vi "ui add or modify exif data.vi"() -> ()   [LabVIEW 2023]
panel:
  out "error":string
  out "Progress":string
  out "Error Array":string[](array[string])
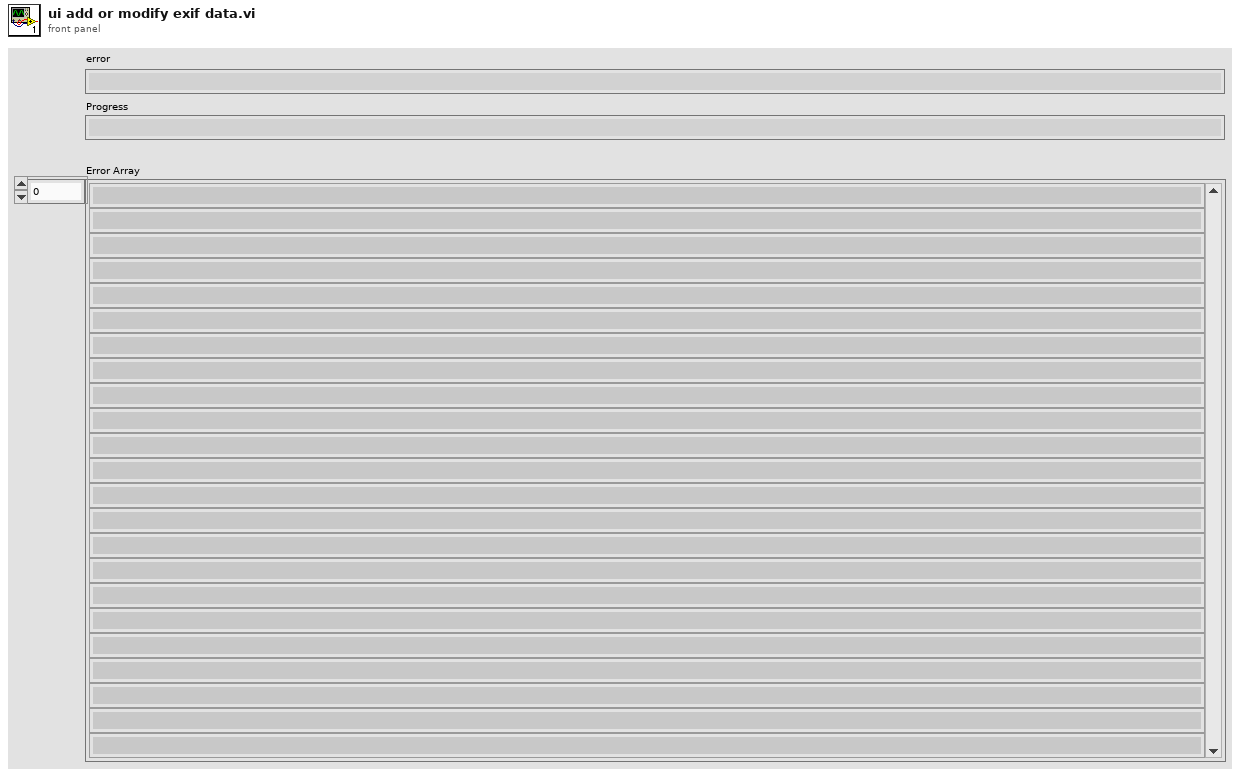
[diagram p1: front panel]
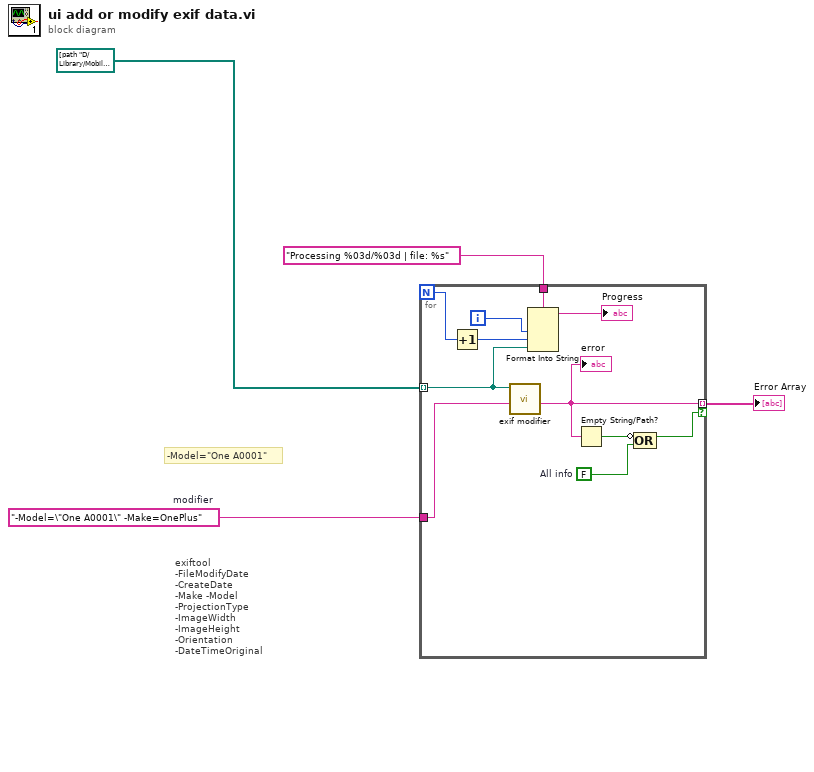
[diagram p0: block diagram]
diagram:
  w4 = "-Model=\"One A0001\" -Make=OnePlus"  # modifier
  # "-Model=\"One A0001\""
  # "exiftool \n-FileModifyDate \n-CreateDate \n-Make -Model \n-ProjectionType \n-ImageWidth \n-ImageHeight \n-Orientation \n-DateTimeOriginal"
  n1 = for {
    N -> [w10]
    tunnel: path[] [path "D:/Library/Mobile Repository/OnePlus1 Data/DNG Files/IMG_20160511_193852.dng", path "D:/Library/Mobile Repository/OnePlus1 Data/DNG Files/IMG_20160511_193916.dng", path "D:/Library/Mobile Repository/OnePlus1 Data/DNG Files/IMG_20160512_134053.dng", path "D:/Library/Mobile Repository/OnePlus1 Data/DNG Files/IMG_20160512_134058.dng", path "D:/Library/Mobile Repository/OnePlus1 Data/DNG Files/IMG_20160512_211940.dng", path "D:/Library/Mobile Repository/OnePlus1 Data/DNG Files/IMG_20160513_183751.dng", path "D:/Library/Mobile Repository/OnePlus1 Data/DNG Files/IMG_20160513_183754.dng", path "D:/Library/Mobile Repository/OnePlus1 Data/DNG Files/IMG_20160513_183809.dng", path "D:/Library/Mobile Repository/OnePlus1 Data/DNG Files/IMG_20160513_183823.dng", path "D:/Library/Mobile Repository/OnePlus1 Data/DNG Files/IMG_20160513_183826.dng", path "D:/Library/Mobile Repository/OnePlus1 Data/DNG Files/IMG_20160513_183840.dng", path "D:/Library/Mobile Repository/OnePlus1 Data/DNG Files/IMG_20160515_153030.dng", path "D:/Library/Mobile Repository/OnePlus1 Data/DNG Files/IMG_20160515_155700.dng", path "D:/Library/Mobile Repository/OnePlus1 Data/DNG Files/IMG_20160516_195620.dng", path "D:/Library/Mobile Repository/OnePlus1 Data/DNG Files/IMG_20160516_195635.dng", path "D:/Library/Mobile Repository/OnePlus1 Data/DNG Files/IMG_20160625_125528.dng", path "D:/Library/Mobile Repository/OnePlus1 Data/DNG Files/IMG_20160625_181705.dng", path "D:/Library/Mobile Repository/OnePlus1 Data/DNG Files/IMG_20160625_181731.dng", path "D:/Library/Mobile Repository/OnePlus1 Data/DNG Files/IMG_20160626_165512.dng", path "D:/Library/Mobile Repository/OnePlus1 Data/DNG Files/IMG_20160626_165517.dng", path "D:/Library/Mobile Repository/OnePlus1 Data/DNG Files/IMG_20160626_165523.dng", path "D:/Library/Mobile Repository/OnePlus1 Data/DNG Files/IMG_20160626_175208.dng", path "D:/Library/Mobile Repository/OnePlus1 Data/DNG Files/IMG_20160626_175216.dng", path "D:/Library/Mobile Repository/OnePlus1 Data/DNG Files/IMG_20160627_101057.dng", path "D:/Library/Mobile Repository/OnePlus1 Data/DNG Files/IMG_20160627_164656.dng", path "D:/Library/Mobile Repository/OnePlus1 Data/DNG Files/IMG_20160627_164716.dng", path "D:/Library/Mobile Repository/OnePlus1 Data/DNG Files/IMG_20160628_173946.dng", path "D:/Library/Mobile Repository/OnePlus1 Data/DNG Files/IMG_20160628_174006.dng", path "D:/Library/Mobile Repository/OnePlus1 Data/DNG Files/IMG_20160628_180806.dng", path "D:/Library/Mobile Repository/OnePlus1 Data/DNG Files/IMG_20160701_175603.dng", path "D:/Library/Mobile Repository/OnePlus1 Data/DNG Files/IMG_20160701_175626.dng", path "D:/Library/Mobile Repository/OnePlus1 Data/DNG Files/IMG_20160703_112526.dng", path "D:/Library/Mobile Repository/OnePlus1 Data/DNG Files/IMG_20160703_113117.dng", path "D:/Library/Mobile Repository/OnePlus1 Data/DNG Files/IMG_20160703_113126.dng", path "D:/Library/Mobile Repository/OnePlus1 Data/DNG Files/IMG_20160703_113144.dng", path "D:/Library/Mobile Repository/OnePlus1 Data/DNG Files/IMG_20160704_184550.dng", path "D:/Library/Mobile Repository/OnePlus1 Data/DNG Files/IMG_20160704_184615.dng", path "D:/Library/Mobile Repository/OnePlus1 Data/DNG Files/IMG_20160704_184624.dng", path "D:/Library/Mobile Repository/OnePlus1 Data/DNG Files/IMG_20160704_184635.dng", path "D:/Library/Mobile Repository/OnePlus1 Data/DNG Files/IMG_20160704_184640.dng", path "D:/Library/Mobile Repository/OnePlus1 Data/DNG Files/IMG_20160705_101728.dng", path "D:/Library/Mobile Repository/OnePlus1 Data/DNG Files/IMG_20160711_080358.dng", path "D:/Library/Mobile Repository/OnePlus1 Data/DNG Files/IMG_20160711_194035.dng", path "D:/Library/Mobile Repository/OnePlus1 Data/DNG Files/IMG_20160712_193401.dng", path "D:/Library/Mobile Repository/OnePlus1 Data/DNG Files/IMG_20160712_193413.dng", path "D:/Library/Mobile Repository/OnePlus1 Data/DNG Files/IMG_20160714_140116.dng", path "D:/Library/Mobile Repository/OnePlus1 Data/DNG Files/IMG_20160714_213325.dng", path "D:/Library/Mobile Repository/OnePlus1 Data/DNG Files/IMG_20160716_173844.dng", path "D:/Library/Mobile Repository/OnePlus1 Data/DNG Files/IMG_20160716_173859.dng", path "D:/Library/Mobile Repository/OnePlus1 Data/DNG Files/IMG_20160716_173910.dng", path "D:/Library/Mobile Repository/OnePlus1 Data/DNG Files/IMG_20160717_163610.dng", path "D:/Library/Mobile Repository/OnePlus1 Data/DNG Files/IMG_20160717_171847.dng", path "D:/Library/Mobile Repository/OnePlus1 Data/DNG Files/IMG_20160717_171851.dng", path "D:/Library/Mobile Repository/OnePlus1 Data/DNG Files/IMG_20160717_171854.dng", path "D:/Library/Mobile Repository/OnePlus1 Data/DNG Files/IMG_20160717_171857.dng", path "D:/Library/Mobile Repository/OnePlus1 Data/DNG Files/IMG_20160717_173333.dng", path "D:/Library/Mobile Repository/OnePlus1 Data/DNG Files/IMG_20160717_174427.dng", path "D:/Library/Mobile Repository/OnePlus1 Data/DNG Files/IMG_20160717_174438.dng", path "D:/Library/Mobile Repository/OnePlus1 Data/DNG Files/IMG_20160718_133800.dng", path "D:/Library/Mobile Repository/OnePlus1 Data/DNG Files/IMG_20160718_194912.dng", path "D:/Library/Mobile Repository/OnePlus1 Data/DNG Files/IMG_20160719_223735.dng", path "D:/Library/Mobile Repository/OnePlus1 Data/DNG Files/IMG_20160719_223748.dng", path "D:/Library/Mobile Repository/OnePlus1 Data/DNG Files/IMG_20160719_223758.dng", path "D:/Library/Mobile Repository/OnePlus1 Data/DNG Files/IMG_20160720_180640.dng", path "D:/Library/Mobile Repository/OnePlus1 Data/DNG Files/IMG_20160722_132434.dng", path "D:/Library/Mobile Repository/OnePlus1 Data/DNG Files/IMG_20160722_132456.dng", path "D:/Library/Mobile Repository/OnePlus1 Data/DNG Files/IMG_20160722_165004.dng", path "D:/Library/Mobile Repository/OnePlus1 Data/DNG Files/IMG_20160722_165020.dng", path "D:/Library/Mobile Repository/OnePlus1 Data/DNG Files/IMG_20160723_175249.dng", path "D:/Library/Mobile Repository/OnePlus1 Data/DNG Files/IMG_20160723_194201.dng", path "D:/Library/Mobile Repository/OnePlus1 Data/DNG Files/IMG_20160724_125207.dng", path "D:/Library/Mobile Repository/OnePlus1 Data/DNG Files/IMG_20160727_181230.dng", path "D:/Library/Mobile Repository/OnePlus1 Data/DNG Files/IMG_20160729_144139.dng", path "D:/Library/Mobile Repository/OnePlus1 Data/DNG Files/IMG_20160729_144143.dng", path "D:/Library/Mobile Repository/OnePlus1 Data/DNG Files/IMG_20160729_144445.dng", path "D:/Library/Mobile Repository/OnePlus1 Data/DNG Files/IMG_20160729_144447.dng", path "D:/Library/Mobile Repository/OnePlus1 Data/DNG Files/IMG_20160729_144454.dng", path "D:/Library/Mobile Repository/OnePlus1 Data/DNG Files/IMG_20160729_144522.dng", path "D:/Library/Mobile Repository/OnePlus1 Data/DNG Files/IMG_20160729_144617.dng", path "D:/Library/Mobile Repository/OnePlus1 Data/DNG Files/IMG_20160729_144621.dng", path "D:/Library/Mobile Repository/OnePlus1 Data/DNG Files/IMG_20160729_144700.dng", path "D:/Library/Mobile Repository/OnePlus1 Data/DNG Files/IMG_20160729_144705.dng", path "D:/Library/Mobile Repository/OnePlus1 Data/DNG Files/IMG_20160729_144732.dng", path "D:/Library/Mobile Repository/OnePlus1 Data/DNG Files/IMG_20160729_145926.dng", path "D:/Library/Mobile Repository/OnePlus1 Data/DNG Files/IMG_20160729_145931.dng", path "D:/Library/Mobile Repository/OnePlus1 Data/DNG Files/IMG_20160729_145933.dng", path "D:/Library/Mobile Repository/OnePlus1 Data/DNG Files/IMG_20160730_200730.dng", path "D:/Library/Mobile Repository/OnePlus1 Data/DNG Files/IMG_20160730_201515.dng", path "D:/Library/Mobile Repository/OnePlus1 Data/DNG Files/IMG_20160730_202503.dng", path "D:/Library/Mobile Repository/OnePlus1 Data/DNG Files/IMG_20160730_202742.dng", path "D:/Library/Mobile Repository/OnePlus1 Data/DNG Files/IMG_20160730_203522.dng", path "D:/Library/Mobile Repository/OnePlus1 Data/DNG Files/IMG_20160730_203529.dng", path "D:/Library/Mobile Repository/OnePlus1 Data/DNG Files/IMG_20160802_184843.dng", path "D:/Library/Mobile Repository/OnePlus1 Data/DNG Files/IMG_20160802_184858.dng", path "D:/Library/Mobile Repository/OnePlus1 Data/DNG Files/IMG_20160802_184916.dng", path "D:/Library/Mobile Repository/OnePlus1 Data/DNG Files/IMG_20160802_184928.dng", path "D:/Library/Mobile Repository/OnePlus1 Data/DNG Files/IMG_20160802_185052.dng", path "D:/Library/Mobile Repository/OnePlus1 Data/DNG Files/IMG_20160802_185127.dng", path "D:/Library/Mobile Repository/OnePlus1 Data/DNG Files/IMG_20160802_185156.dng", path "D:/Library/Mobile Repository/OnePlus1 Data/DNG Files/IMG_20160807_204018.dng", path "D:/Library/Mobile Repository/OnePlus1 Data/DNG Files/IMG_20160807_204023.dng", path "D:/Library/Mobile Repository/OnePlus1 Data/DNG Files/IMG_20160807_204029.dng", path "D:/Library/Mobile Repository/OnePlus1 Data/DNG Files/IMG_20160807_204033.dng", path "D:/Library/Mobile Repository/OnePlus1 Data/DNG Files/IMG_20160807_204037.dng", path "D:/Library/Mobile Repository/OnePlus1 Data/DNG Files/IMG_20160807_204044.dng", path "D:/Library/Mobile Repository/OnePlus1 Data/DNG Files/IMG_20160807_204053.dng", path "D:/Library/Mobile Repository/OnePlus1 Data/DNG Files/IMG_20160807_204106.dng", path "D:/Library/Mobile Repository/OnePlus1 Data/DNG Files/IMG_20160807_204114.dng", path "D:/Library/Mobile Repository/OnePlus1 Data/DNG Files/IMG_20160807_204119.dng", path "D:/Library/Mobile Repository/OnePlus1 Data/DNG Files/IMG_20160807_204123.dng", path "D:/Library/Mobile Repository/OnePlus1 Data/DNG Files/IMG_20160807_204126.dng", path "D:/Library/Mobile Repository/OnePlus1 Data/DNG Files/IMG_20160807_204128.dng", path "D:/Library/Mobile Repository/OnePlus1 Data/DNG Files/IMG_20160810_092958.dng", path "D:/Library/Mobile Repository/OnePlus1 Data/DNG Files/IMG_20160810_093025.dng", path "D:/Library/Mobile Repository/OnePlus1 Data/DNG Files/IMG_20160810_171857.dng", path "D:/Library/Mobile Repository/OnePlus1 Data/DNG Files/IMG_20160810_171909.dng", path "D:/Library/Mobile Repository/OnePlus1 Data/DNG Files/IMG_20160812_165342.dng", path "D:/Library/Mobile Repository/OnePlus1 Data/DNG Files/IMG_20160812_165347.dng", path "D:/Library/Mobile Repository/OnePlus1 Data/DNG Files/IMG_20160812_165353.dng", path "D:/Library/Mobile Repository/OnePlus1 Data/DNG Files/IMG_20160812_165358.dng", path "D:/Library/Mobile Repository/OnePlus1 Data/DNG Files/IMG_20160812_165408.dng", path "D:/Library/Mobile Repository/OnePlus1 Data/DNG Files/IMG_20160812_165416.dng", path "D:/Library/Mobile Repository/OnePlus1 Data/DNG Files/IMG_20160812_165813.dng", path "D:/Library/Mobile Repository/OnePlus1 Data/DNG Files/IMG_20160812_165823.dng", path "D:/Library/Mobile Repository/OnePlus1 Data/DNG Files/IMG_20160813_114335.dng", path "D:/Library/Mobile Repository/OnePlus1 Data/DNG Files/IMG_20160813_114822.dng", path "D:/Library/Mobile Repository/OnePlus1 Data/DNG Files/IMG_20160813_114827.dng", path "D:/Library/Mobile Repository/OnePlus1 Data/DNG Files/IMG_20160813_115020.dng", path "D:/Library/Mobile Repository/OnePlus1 Data/DNG Files/IMG_20160814_102219.dng", path "D:/Library/Mobile Repository/OnePlus1 Data/DNG Files/IMG_20160814_191707.dng", path "D:/Library/Mobile Repository/OnePlus1 Data/DNG Files/IMG_20160815_204403.dng", path "D:/Library/Mobile Repository/OnePlus1 Data/DNG Files/IMG_20160816_110056.dng", path "D:/Library/Mobile Repository/OnePlus1 Data/DNG Files/IMG_20160816_192912.dng", path "D:/Library/Mobile Repository/OnePlus1 Data/DNG Files/IMG_20160816_211622.dng", path "D:/Library/Mobile Repository/OnePlus1 Data/DNG Files/IMG_20160816_211633.dng", path "D:/Library/Mobile Repository/OnePlus1 Data/DNG Files/IMG_20160819_170033.dng", path "D:/Library/Mobile Repository/OnePlus1 Data/DNG Files/IMG_20160819_170038.dng", path "D:/Library/Mobile Repository/OnePlus1 Data/DNG Files/IMG_20160819_170041.dng", path "D:/Library/Mobile Repository/OnePlus1 Data/DNG Files/IMG_20160820_081503.dng", path "D:/Library/Mobile Repository/OnePlus1 Data/DNG Files/IMG_20160820_134938.dng", path "D:/Library/Mobile Repository/OnePlus1 Data/DNG Files/IMG_20160820_150631.dng", path "D:/Library/Mobile Repository/OnePlus1 Data/DNG Files/IMG_20160823_143226.dng", path "D:/Library/Mobile Repository/OnePlus1 Data/DNG Files/IMG_20160826_075543.dng", path "D:/Library/Mobile Repository/OnePlus1 Data/DNG Files/IMG_20160826_124239.dng", path "D:/Library/Mobile Repository/OnePlus1 Data/DNG Files/IMG_20160828_085112.dng", path "D:/Library/Mobile Repository/OnePlus1 Data/DNG Files/IMG_20160828_133108.dng", path "D:/Library/Mobile Repository/OnePlus1 Data/DNG Files/IMG_20160830_090537.dng", path "D:/Library/Mobile Repository/OnePlus1 Data/DNG Files/IMG_20160830_142547.dng", path "D:/Library/Mobile Repository/OnePlus1 Data/DNG Files/IMG_20160830_142611.dng", path "D:/Library/Mobile Repository/OnePlus1 Data/DNG Files/IMG_20160830_142624.dng", path "D:/Library/Mobile Repository/OnePlus1 Data/DNG Files/IMG_20160830_142636.dng", path "D:/Library/Mobile Repository/OnePlus1 Data/DNG Files/IMG_20160831_135831.dng", path "D:/Library/Mobile Repository/OnePlus1 Data/DNG Files/IMG_20160901_073656.dng", path "D:/Library/Mobile Repository/OnePlus1 Data/DNG Files/IMG_20160901_191953.dng", path "D:/Library/Mobile Repository/OnePlus1 Data/DNG Files/IMG_20160902_195552.dng", path "D:/Library/Mobile Repository/OnePlus1 Data/DNG Files/IMG_20160902_195628.dng", path "D:/Library/Mobile Repository/OnePlus1 Data/DNG Files/IMG_20160905_174957.dng", path "D:/Library/Mobile Repository/OnePlus1 Data/DNG Files/IMG_20160906_132133.dng", path "D:/Library/Mobile Repository/OnePlus1 Data/DNG Files/IMG_20160906_132303.dng", path "D:/Library/Mobile Repository/OnePlus1 Data/DNG Files/IMG_20160908_075523.dng", path "D:/Library/Mobile Repository/OnePlus1 Data/DNG Files/IMG_20160909_130311.dng", path "D:/Library/Mobile Repository/OnePlus1 Data/DNG Files/IMG_20160909_191224.dng", path "D:/Library/Mobile Repository/OnePlus1 Data/DNG Files/IMG_20160909_191233.dng", path "D:/Library/Mobile Repository/OnePlus1 Data/DNG Files/IMG_20160911_094414.dng", path "D:/Library/Mobile Repository/OnePlus1 Data/DNG Files/IMG_20160911_095926.dng", path "D:/Library/Mobile Repository/OnePlus1 Data/DNG Files/IMG_20160911_115344.dng", path "D:/Library/Mobile Repository/OnePlus1 Data/DNG Files/IMG_20160914_182328.dng", path "D:/Library/Mobile Repository/OnePlus1 Data/DNG Files/IMG_20160914_182332.dng", path "D:/Library/Mobile Repository/OnePlus1 Data/DNG Files/IMG_20160914_182335.dng", path "D:/Library/Mobile Repository/OnePlus1 Data/DNG Files/IMG_20160914_182340.dng", path "D:/Library/Mobile Repository/OnePlus1 Data/DNG Files/IMG_20160914_182344.dng", path "D:/Library/Mobile Repository/OnePlus1 Data/DNG Files/IMG_20160914_182358.dng", path "D:/Library/Mobile Repository/OnePlus1 Data/DNG Files/IMG_20160914_182406.dng", path "D:/Library/Mobile Repository/OnePlus1 Data/DNG Files/IMG_20160915_085931.dng", path "D:/Library/Mobile Repository/OnePlus1 Data/DNG Files/IMG_20160915_085955.dng", path "D:/Library/Mobile Repository/OnePlus1 Data/DNG Files/IMG_20160919_144856.dng", path "D:/Library/Mobile Repository/OnePlus1 Data/DNG Files/IMG_20160919_145004.dng", path "D:/Library/Mobile Repository/OnePlus1 Data/DNG Files/IMG_20160919_145925.dng", path "D:/Library/Mobile Repository/OnePlus1 Data/DNG Files/IMG_20160921_141024.dng", path "D:/Library/Mobile Repository/OnePlus1 Data/DNG Files/IMG_20160921_141849.dng", path "D:/Library/Mobile Repository/OnePlus1 Data/DNG Files/IMG_20160921_142257.dng", path "D:/Library/Mobile Repository/OnePlus1 Data/DNG Files/IMG_20160921_142309.dng", path "D:/Library/Mobile Repository/OnePlus1 Data/DNG Files/IMG_20160924_181417.dng", path "D:/Library/Mobile Repository/OnePlus1 Data/DNG Files/IMG_20160925_115454.dng", path "D:/Library/Mobile Repository/OnePlus1 Data/DNG Files/IMG_20160925_115523.dng", path "D:/Library/Mobile Repository/OnePlus1 Data/DNG Files/IMG_20160925_115802.dng", path "D:/Library/Mobile Repository/OnePlus1 Data/DNG Files/IMG_20170204_170536.dng", path "D:/Library/Mobile Repository/OnePlus1 Data/DNG Files/IMG_20170204_173243.dng", path "D:/Library/Mobile Repository/OnePlus1 Data/DNG Files/IMG_20170204_175123.dng", path "D:/Library/Mobile Repository/OnePlus1 Data/DNG Files/IMG_20170204_175147.dng", path "D:/Library/Mobile Repository/OnePlus1 Data/DNG Files/IMG_20170204_175203.dng", path "D:/Library/Mobile Repository/OnePlus1 Data/DNG Files/IMG_20170204_180510.dng", path "D:/Library/Mobile Repository/OnePlus1 Data/DNG Files/IMG_20170204_180624.dng", path "D:/Library/Mobile Repository/OnePlus1 Data/DNG Files/IMG_20170204_180629.dng", path "D:/Library/Mobile Repository/OnePlus1 Data/DNG Files/IMG_20170204_180700.dng", path "D:/Library/Mobile Repository/OnePlus1 Data/DNG Files/IMG_20170224_201238.dng"] ("All Files in Dir") -> [w7] mode=indexing
    tunnel: w4 -> [w15]
    tunnel: [w6] -> w3 mode=indexing if=w13
    tunnel: "Processing %03d/%03d | file: %s" ("String") -> [w9]
    i -> [w11]
    w12 = FALSE  # All info
    n2 = Increment(x=w10) -> (x+1=w5:i32)
    n3 = call "exif modifier.vi"("modifier"=w15, "input 1"=w7) -> ("error"=w6:string)  [unwired: 9 in]
    "error" <- w6
    n4 = Format Into String(format string=w9, w11, w5, w7) -> (resulting string=→"Progress":string)  [unwired: 2 in, 1 out]
    n5 = Empty String/Path?(string/path=w6) -> (empty?=w14:bool)
    n6 = Compound Arithmetic op=OR(invert w14, w12) -> (w13:bool)
  }
  "Error Array" <- w3
